vi "Public SV.vi"(8 "error in (no error)":errorcluster, 11 "NeedleValve in":refnum<class "NeedleValve.lvclass">) -> (0 "error out":errorcluster, 3 "NeedleValve out":refnum<class "NeedleValve.lvclass">)   [LabVIEW 2019, in "NeedleValve.lvclass"]
uses:
  NeedleValve.lvclass
  D:/GIT H4000/H4000/src/Device_class/Device.lvclass
  D:/GIT H4000/H4000/src/Proccess_class/Proccess.lvclass
  Proccess_class/Proccess.lvclass/Proccess.ctl
  Device_class/Device.lvclass/Device.ctl
  NeedleValve.lvclass/NeedleValve.ctl
  SV_Puplisher_class/SV_Publisher.lvclass/SV_Publisher.ctl
  SV_Puplisher_class/Set SV.vi/1ae5d02c-efd0-450a-8aa4-8388e25d05bc.vi
  SV_Puplisher_class/SV_Publisher.lvclass
  Proccess_class/Proccess.lvclass
  Device_class/Device.lvclass
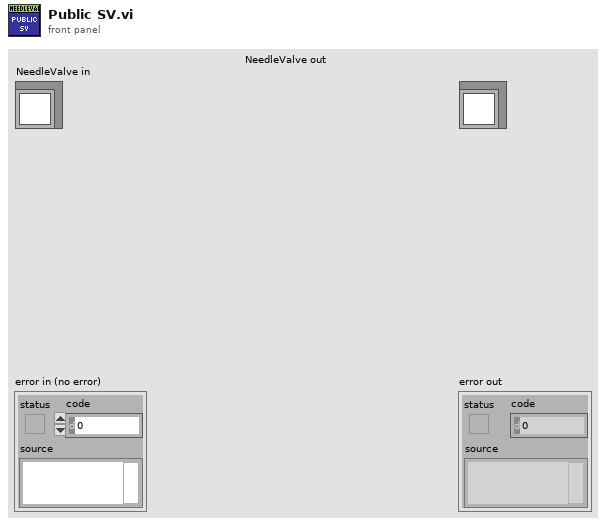
[diagram p1: front panel]
types:
  T1 = typedef "Needle Valve Settings.ctl" = cluster{"average size":i32, "open force":u16, "close force":u16, "open settings":T2, "close settings":T2, "Offset angle":dbl, "Start angle":dbl}
  T2 = typedef "MB_ENGINE.lvclass/Settings.ctl" = cluster{"ACC Steps Per Sec^2":u16, "DEC Steps Per Sec^2":u16, "Min Velosity Step Per Sec":u16, "Max Velosity Step Per Sec":u16, "MicroStep":u16}
  T3 = typedef "Proccess.lvclass/TAGs.ctl" = cluster{"TAG":string, "PTAG":string, "DESC":string}
  T4 = typedef "Needle Valve Data.ctl" = cluster{"Engine State":T5, "StateValveModbus":T6, "Alarms":T7, "RAW":i32, "Angele":dbl, "Step":i32, "Encoder":i32, "Kinematic":T2, "Limits":T8, "EncoderMax":i32, "Counter Max Dont Update":i32, "EncoderMin":i32, "Counter Min Dont Update":i32, "Prepere Counter":i32, "STEP INIT":i32, "offset - Angel":dbl}
  T5 = typedef "MB_ENGINE.lvclass/Engine State.ctl" = u16
  T6 = typedef "Needle Valve State.ctl" = enum16{"STOPED", "CLOSED", "OPENED", "OPENING", "CLOSING", "FULL_CLOSE", "PREP_OPEN"}
  T7 = typedef "MB_ENGINE.lvclass/Engine Alarms.ctl" = cluster{"OL":bool, "TF":bool, "STL":bool, "OCP":bool, "CPUV":bool, "UVLO":bool, "SPI_ERROR":bool, "Fault":bool, "OL 2":bool, "TF 2":bool, "STL 2":bool, "OCP 2":bool, "CPUV 2":bool, "UVLO 2":bool, "reserved":bool, "InitDone":bool}
  T8 = typedef "MB_ENGINE.lvclass/Limits Status.ctl" = cluster{"Fault 2 Switch":bool, "Fault 1 Switch":bool, "Center(Home)":bool, "Lower Limit":bool, "Upper Limit":bool}
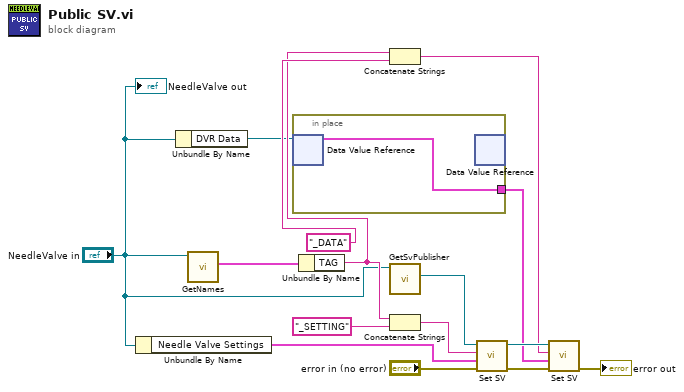
[diagram p0: block diagram]
diagram:
  n1 = Unbundle By Name("NeedleValve in") -> ("Needle Valve Settings"=w5:T1)
  n2 = Unbundle By Name("NeedleValve in") -> ("DVR Data"=w2:refnum<data-value>)
  n3 = call "GetNames.vi"("Proccess in"="NeedleValve in") -> ("Tags"=w8:T3)  [unwired: 10 in]
  n4 = in-place {
    in-place-border: [w16] -> w1
    n5 = in-place-dvr #1(w2) -> (w16:T4)  [unwired: 1 out]
    n6 = in-place-dvr #1() -> ()  [unwired: 1 in, 2 out]
  }
  n7 = Unbundle By Name(w8) -> ("TAG"=w7:string)
  n8 = Concatenate Strings(w7, "_DATA" ("string")) -> (w4:string)
  n9 = call "GetSvPublisher.vi"("Device in"="NeedleValve in") -> ("SV_Publisher.lvclass"=w13:refnum<class "SV_Publisher.lvclass">)  [unwired: 10 in]
  n10 = Concatenate Strings(w7, "_SETTING" ("SV Name")) -> (w6:string)
  n11 = call "Set SV.vi"("error in (no error)"="error in (no error)", "SV Value"=w5, "SV Name"=w6, "SV_Publisher in"=w13) -> ("error out"=w11:errorcluster, "SV_Publisher out"=w10:refnum<class "SV_Publisher.lvclass">)  [unwired: 6 in]
  n12 = call "Set SV.vi"("error in (no error)"=w11, "SV Value"=w1, "SV Name"=w4, "SV_Publisher in"=w10) -> ("error out"=→"error out":errorcluster)  [unwired: 6 in, 1 out]
  "NeedleValve out" <- "NeedleValve in"
